vi "Calc Conf.vi"(8 "error in (no error)":errorcluster, 11 "data":sgl[](array[numeric])) -> (0 "error out":errorcluster, 2 "result":cluster{"conf":sgl, "class":string}[](array[cluster]), 3 "conf":sgl[](array[numeric]))   [LabVIEW 2017, in "process_EfficientNet_B4.lvlib"]
uses:
  process_EfficientNet_B4.lvlib
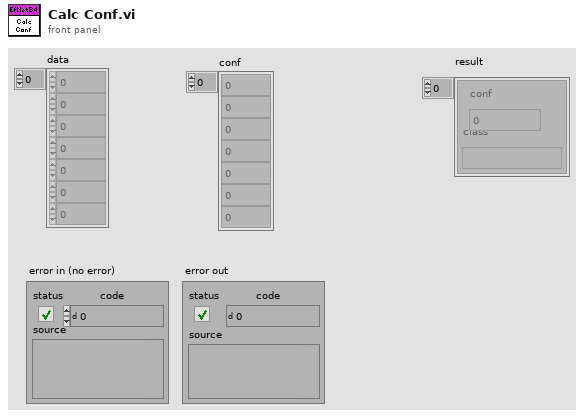
[diagram p1: front panel]
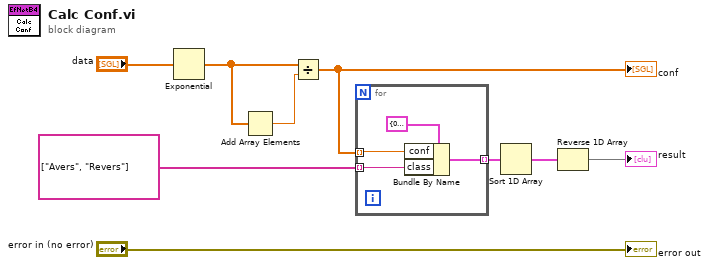
[diagram p0: block diagram]
diagram:
  n1 = Exponential(1:"data") -> (0:w7:sgl[])
  n2 = Add Array Elements(numeric array=w7) -> (sum=w6:sgl)
  n3 = Divide(x=w7, y=w6) -> (x/y=w5:sgl[])
  "conf" <- w5
  n4 = for {
    tunnel: w5 -> [w13] mode=indexing
    tunnel: string[] ["Avers", "Revers"] -> [w11] mode=indexing
    tunnel: [w10] -> w3 mode=indexing
    n5 = Bundle By Name(cluster=cluster{"conf":sgl, "class":string} {"conf"=0.0, "class"=""} ("input cluster"), "conf"=w13, "class"=w11) -> (w10:cluster{"conf":sgl, "class":string})
  }
  n6 = Sort 1D Array(array=w3) -> (sorted array=w2:cluster{"conf":sgl, "class":string}[])
  n7 = Reverse 1D Array(array=w2) -> (reversed array=→"result":cluster{"conf":sgl, "class":string}[])
  "error out" <- "error in (no error)"
